vi "Create Plugin.vi"(8 "error in":errorcluster, 11 "configuration":T1) -> (0 "error out":errorcluster)   [LabVIEW 2021, in "InstrumentStudio Plug-In Editor.lvlib"]
uses:
  InstrumentStudio Plug-In Editor.lvlib
  Plugin Configuration.ctl
  Error Strings Global Internal.vi
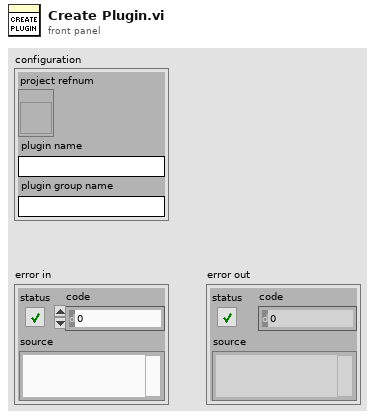
[diagram p1: front panel]
types:
  T1 = typedef "InstrumentStudio Plug-In Editor.lvlib/Plugin Configuration.ctl" = cluster{"project refnum":refnum<vi>, "plugin name":string, "plugin group name":string}
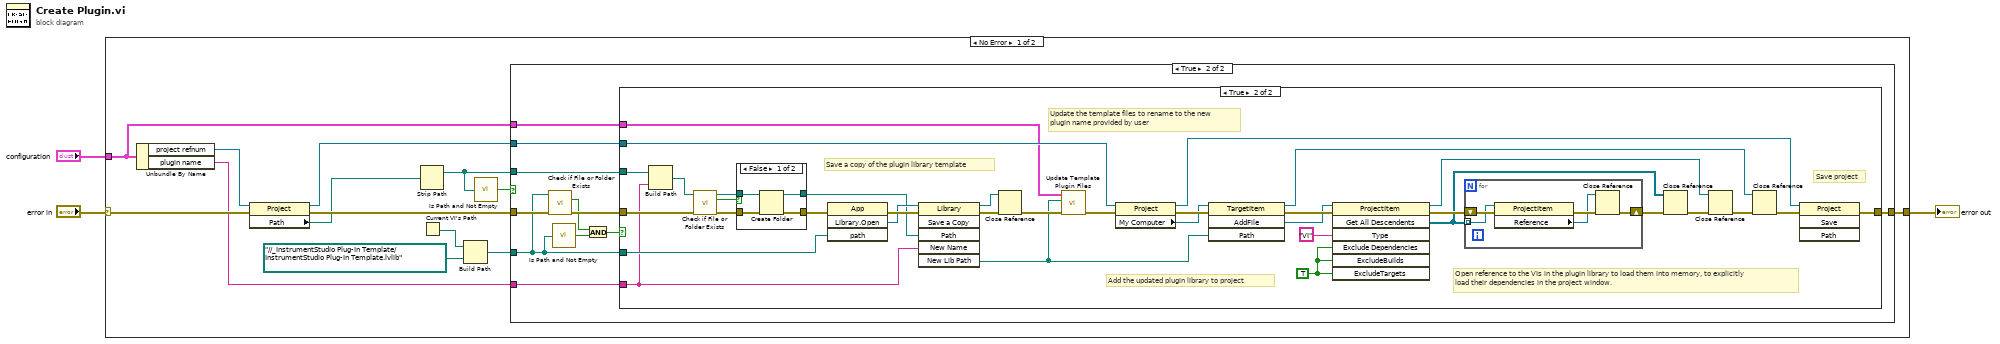
[diagram p0: block diagram]
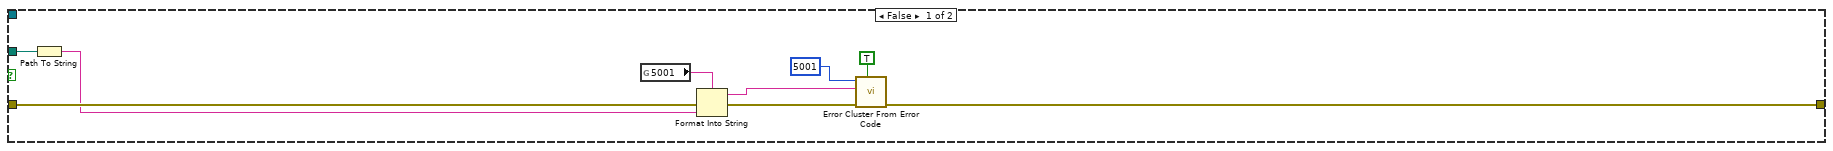
[diagram p2: hidden frame]
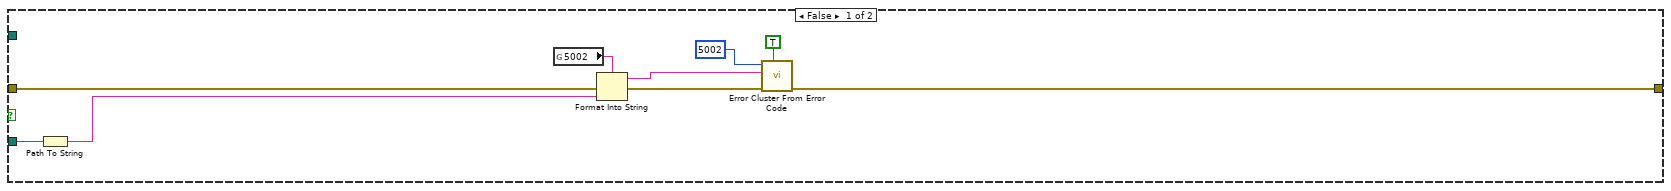
[diagram p3: hidden frame]
diagram:
  n1 = case shown="No Error" "error in" {
    selector: "error in" -> [w13 w92]
    tunnel: "configuration" -> [w15 _]
    tunnel: [w4 w92] -> w1
    frame No Error {
      n2 = Unbundle By Name(w15) -> ("project refnum"=w16:refnum<vi>, "plugin name"=w10:string)
      n3 = property class="Project"(reference=w16, error in=w13) -> (reference out=w14:refnum<vi>, error out=w12:errorcluster, "Path"=w7:path)
      n4 = Strip Path(path=w7) -> (stripped path=w6:path)  [unwired: 1 out]
      n5 = Current VI's Path() -> (path=w9:path)
      n6 = Build Path(base path=w9, name or relative path=path "../../_InstrumentStudio Plug-In Template/InstrumentStudio Plug-In Template.lvlib") -> (appended path=w11:path)
      n7 = call <vilib>:"Is Path and Not Empty.vi"("path"=w6) -> ("Is Path and Not Empty?"=w5:bool)  [unwired: 4 in]
      n8 = case shown="True" w5 {
        tunnel: w6 -> [w19 w36]
        tunnel: w15 -> [_ w35]
        tunnel: w14 -> [_ w34]
        tunnel: w12 -> [w21 w33]
        tunnel: [w22 w32] -> w4
        tunnel: w11 -> [_ w26]
        tunnel: w10 -> [_ w30]
        frame False {
          n9 = Path To String(path=w19) -> (string=w20:string)
          n10 = global read "Error Strings Global Internal.vi" "5001"() -> (w23:string)
          n11 = Format Into String(format string=w23, error in=w21, w20) -> (resulting string=w24:string, error out=w25:errorcluster)  [unwired: 1 in]
          n12 = call <vilib>:"Error Cluster From Error Code.vi"("show call chain? (False)"=TRUE, "error in (no error)"=w25, "error message (\"\")"=w24, "error code (0)"=5001) -> ("error out"=w22:errorcluster)  [unwired: 5 in]
        }
        frame True {
          n13 = call <vilib>:"Check if File or Folder Exists.vi"("error in (no error)"=w33, "path"=w26) -> ("error out"=w31:errorcluster, "file or folder exists?"=w28:bool)  [unwired: 7 in, 1 out]
          n14 = call <vilib>:"Is Path and Not Empty.vi"("path"=w26) -> ("Is Path and Not Empty?"=w29:bool)  [unwired: 4 in]
          n15 = And(x=w28, y=w29) -> (x .and. y?=w27:bool)
          n16 = case shown="True" w27 {
            tunnel: w36 -> [_ w69]
            tunnel: w35 -> [_ w62]
            tunnel: w34 -> [_ w64]
            tunnel: w31 -> [w44 w71]
            tunnel: [w43 w65] -> w32
            tunnel: w26 -> [w39 w59]
            tunnel: w30 -> [_ w58]
            frame False {
              n17 = Path To String(path=w39) -> (string=w38:string)
              n18 = global read "Error Strings Global Internal.vi" "5002"() -> (w41:string)
              n19 = Format Into String(format string=w41, error in=w44, w38) -> (resulting string=w42:string, error out=w45:errorcluster)  [unwired: 1 in]
              n20 = call <vilib>:"Error Cluster From Error Code.vi"("show call chain? (False)"=TRUE, "error in (no error)"=w45, "error message (\"\")"=w42, "error code (0)"=5002) -> ("error out"=w43:errorcluster)  [unwired: 5 in]
            }
            frame True {
              w48 = TRUE ("ExcludeTargets")
              # "Open reference to the VIs in the plugin library to load them into memory, to explicitly\nload their dependencies in the project window."
              # "Save project"
              # "Add the updated plugin library to project"
              # "Update the template files to rename to the new\nplugin name provided by user"
              # "Save a copy of the plugin library template"
              n21 = Build Path(base path=w69, name or relative path=w58) -> (appended path=w70:path)
              n22 = call <vilib>:"Check if File or Folder Exists.vi"("error in (no error)"=w71, "path"=w70) -> ("error out"=w73:errorcluster, "file or folder exists?"=w75:bool, "dup path"=w74:path)  [unwired: 7 in]
              n23 = case shown="False" w75 {
                tunnel: w73 -> [w89 w90]
                tunnel: w74 -> [w88 w91]
                tunnel: [w87 w91] -> w57
                tunnel: [w86 w90] -> w79
                frame False {
                  n24 = Create Folder(path (use dialog)=w88, error in=w89) -> (created path=w87:path, error out=w86:errorcluster)  [unwired: 1 in, 1 out]
                }
                frame True {
                }
              }
              n25 = invoke class="App" method="Library.Open"(error in=w79, "path"=w59) -> (error out=w77:errorcluster, "Open Library"=w72:refnum<vi>)  [unwired: 2 in, 2 out]
              n26 = invoke class="Library" method="Save a Copy"(reference=w72, error in=w77, "Path"=w57, "New Name"=w58) -> (reference out=w76:refnum<vi>, error out=w78:errorcluster, "New Lib Path"=w56:path)  [unwired: 2 in, 3 out]
              n27 = Close Reference(reference=w76, error in (no error)=w78) -> (error out=w63:errorcluster)
              n28 = call "Update Template Plugin Files.vi"("error in"=w63, "plugin library path"=w56, "configuration"=w62) -> ("error out"=w80:errorcluster)  [unwired: 8 in]
              n29 = property class="Project"(reference=w64, error in=w80) -> (reference out=w68:refnum<vi>, error out=w67:errorcluster, "My Computer"=w66:refnum<vi>)
              n30 = invoke class="TargetItem" method="AddFile"(reference=w66, error in=w67, "Path"=w56) -> (reference out=w60:refnum<vi>, error out=w55:errorcluster, "AddFile"=w53:refnum<vi>)  [unwired: 1 in, 1 out]
              n31 = invoke class="ProjectItem" method="Get All Descendents"(reference=w53, error in=w55, "Type"="VI", "Exclude Dependencies"=w48, "ExcludeBuilds"=w48, "ExcludeTargets"=w48) -> (reference out=w49:refnum<vi>, error out=w54:errorcluster, "All Descendents"=w51:refnum<vi>[])  [unwired: 1 in, 4 out]
              n32 = for {
                shift-right: [w81] -> w47
                shift-left: w54 -> [w85]
                tunnel: w51 -> [w83] mode=indexing
                n33 = property class="ProjectItem"(reference=w83, error in=w85) -> (error out=w84:errorcluster, "Reference"=w82:refnum<vi>)  [unwired: 1 out]
                n34 = Close Reference(reference=w82, error in (no error)=w84) -> (error out=w81:errorcluster)
              }
              n35 = Close Reference(reference=w51, error in (no error)=w47) -> (error out=w52:errorcluster)
              n36 = Close Reference(reference=w49, error in (no error)=w52) -> (error out=w50:errorcluster)
              n37 = Close Reference(reference=w60, error in (no error)=w50) -> (error out=w61:errorcluster)
              n38 = invoke class="Project" method="Save"(reference=w68, error in=w61) -> (error out=w65:errorcluster)  [unwired: 2 in, 3 out]
            }
          }
        }
      }
    }
    frame Error {
    }
  }
  "error out" <- w1
